vi "Rolebook_Create.vi"(0 "reference in":refnum<class "Rolebook.lvclass">, 5 "error in (no error)":errorcluster) -> (14 "reference out":refnum<class "Rolebook.lvclass">, 19 "error out":errorcluster)   [LabVIEW 2018, in "Rolebook.lvclass"]
uses:
  Rolebook.lvclass
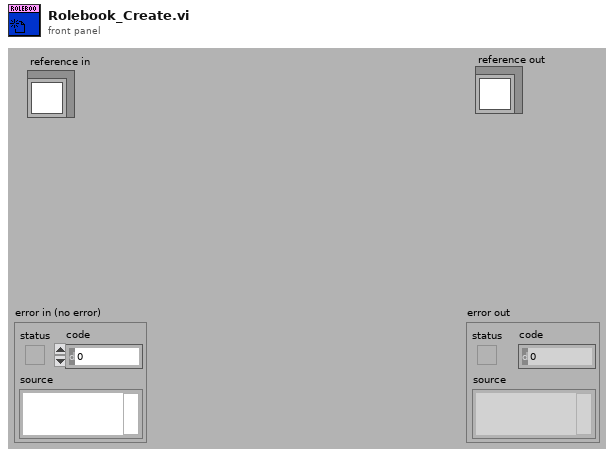
[diagram p1: front panel]
types:
  T1 = typedef "Rolebook.lvclass/ObjectAttributes.ctl" = cluster{"Attribute1":dbl}
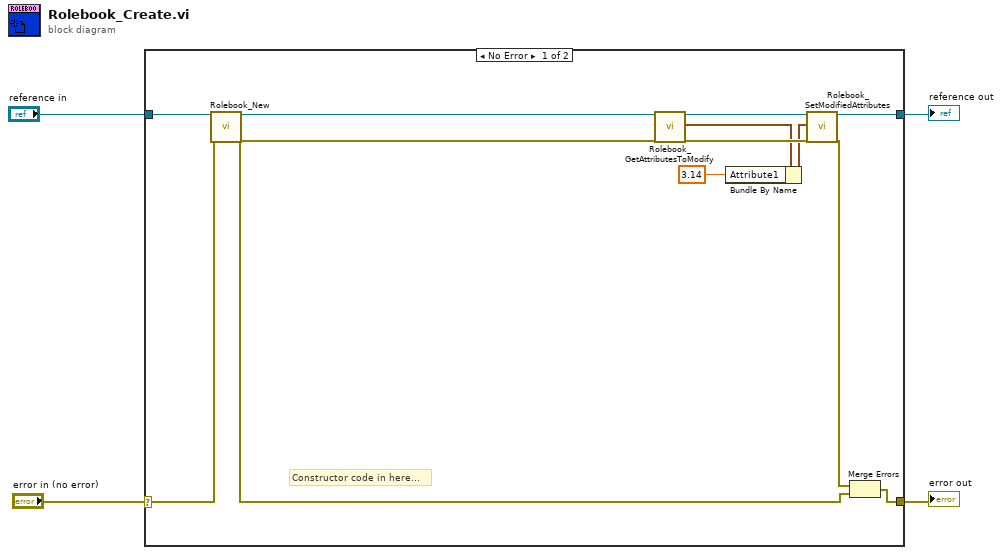
[diagram p0: block diagram]
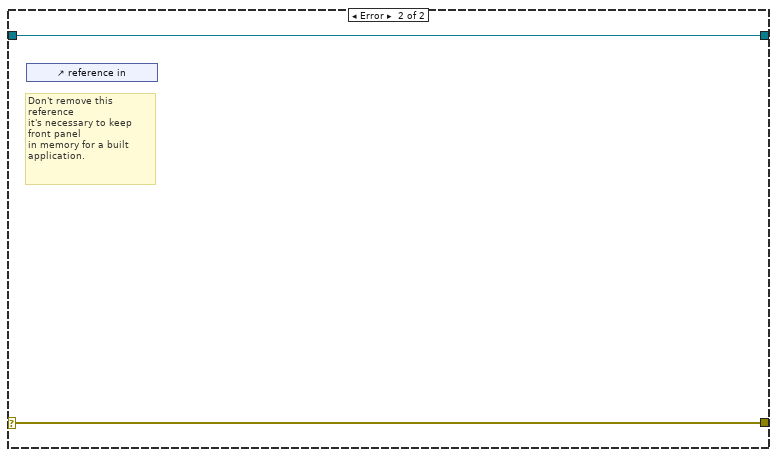
[diagram p2: hidden frame]
diagram:
  n1 = case shown="No Error" "error in (no error)" {
    selector: "error in (no error)" -> [w16 w18]
    tunnel: [w7 w18] -> w4
    tunnel: "reference in" -> [w9 w17]
    tunnel: [w10 w17] -> w2
    frame No Error {
      # "Constructor code in here..."
      n2 = call "Rolebook_New.vi"("reference in"=w9, "error in (no error)"=w16) -> ("reference out"=w8:refnum<class "Rolebook.lvclass">, "error out"=w5:errorcluster)  [unwired: 14 in, 2 out]
      n3 = call "Rolebook_GetAttributesToModify.vi"("reference in"=w8, "error in (no error)"=w5) -> ("reference out"=w14:refnum<class "Rolebook.lvclass">, "Attributes"=w13:T1, "error out"=w15:errorcluster)  [unwired: 14 in, 1 out]
      n4 = Bundle By Name(cluster=w13, "Attribute1"=3.14 ("attribute1")) -> (w12:T1)
      n5 = call "Rolebook_SetModifiedAttributes.vi"("reference in"=w14, "Attributes"=w12, "error in (no error)"=w15) -> ("reference out"=w10:refnum<class "Rolebook.lvclass">, "error out"=w6:errorcluster)  [unwired: 15 in]
      n6 = Merge Errors(w6, w5) -> (w7:errorcluster)
    }
    frame Error {
      # "Don't remove this reference\nit's necessary to keep front panel\nin memory for a built application."
      n7 = control-ref of="reference in"() -> ()  [unwired: 1 out]
    }
  }
  "error out" <- w4
  "reference out" <- w2
